vi "add.vi"(11 "arguments":T1[](array[typedef])) -> (3 "Expression 3":T1)   [LabVIEW 2021]
uses:
  Expression.ctl
  ExpressionType.ctl
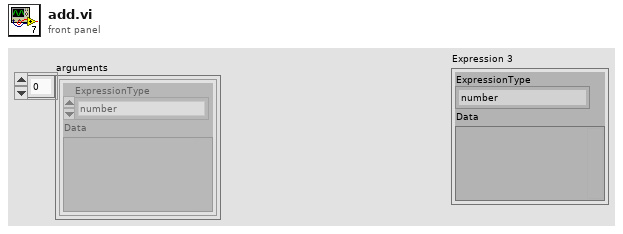
[diagram p1: front panel]
types:
  T1 = typedef "Expression.ctl" = cluster{"ExpressionType":T2, "Data":variant}
  T2 = typedef "ExpressionType.ctl" = enum16{"number", "string", "symbol", "primitive", "list", "closure", "nil", "error"}
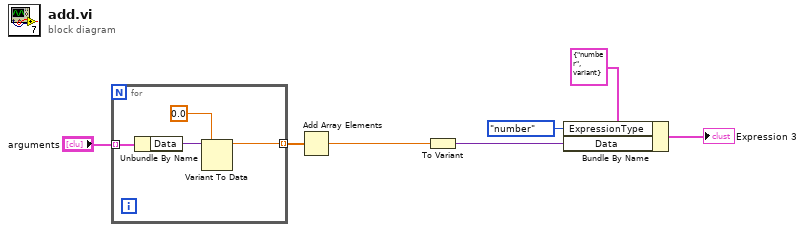
[diagram p0: block diagram]
diagram:
  n1 = for {
    tunnel: "arguments" -> [w11] mode=indexing
    tunnel: [w8] -> w2 mode=indexing
    n2 = Unbundle By Name(w11) -> ("Data"=w10:variant)
    n3 = Variant To Data(type=0.0, Variant=w10) -> (data=w8:dbl)  [unwired: 1 in, 1 out]
  }
  n4 = Add Array Elements(numeric array=w2) -> (sum=w1:dbl)
  n5 = To Variant(anything=w1) -> (Variant=w4:variant)
  n6 = Bundle By Name(cluster=T1 {"ExpressionType"=enum."number", "Data"=variant} ("Expression 3"), "ExpressionType"=ExpressionType."number", "Data"=w4) -> (→"Expression 3":T1)
